vi "Signal List Keys.vi"(8 "error in":errorcluster, 11 "AnalogInput in":refnum<class "AnalogInput.lvclass">) -> (0 "error out":errorcluster, 2 "CFG Signal Headers":string[](array[string]), 3 "AnalogInput out":refnum<class "AnalogInput.lvclass">)   [LabVIEW 2019, in "AnalogInput.lvlib" / "AnalogInput.lvclass"]
uses:
  Library/AnalogInput.lvclass
  Custom Controls/Signal Keys.ctl
  builds/Instruments/Instruments.lvlibp/Library/Instruments.lvclass
panel:
  in  "Signal Keys":T1
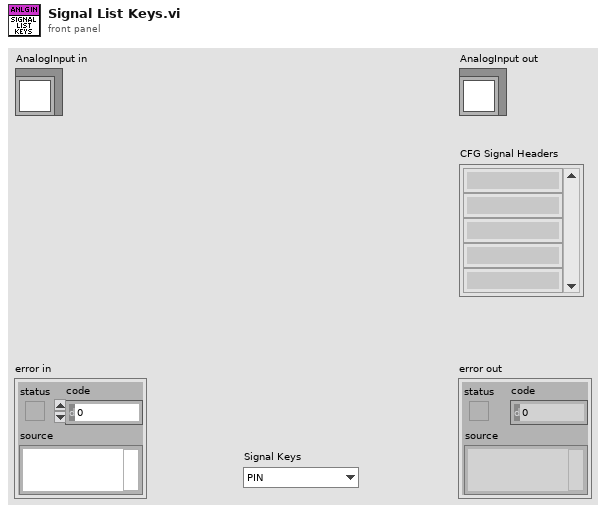
[diagram p1: front panel]
types:
  T1 = typedef "AnalogInput.lvlib/AnalogInput.lvclass/Signal Keys.ctl" = enum16{"PIN", "NAME", "MIN", "MAX", "TRIG_NAME", "TRIG_SRC"}
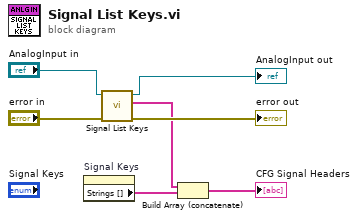
[diagram p0: block diagram]
diagram:
  n1 = property on="Signal Keys" class="Enum (strict)"() -> ("Strings []"=w3:string[])  [unwired: 2 in, 2 out]
  n2 = call-parent "Signal List Keys.vi"("error in"="error in", "Instruments in"="AnalogInput in") -> ("error out"=→"error out":errorcluster, "CFG Signal Headers"=w2:string[], "Instruments out"=→"AnalogInput out":refnum<class "AnalogInput.lvclass">)  [unwired: 7 in]
  n3 = Build Array (concatenate)(w2, w3) -> (→"CFG Signal Headers":string[])
